vi "Handle Error.vi"(8 "error in (no error)":errorcluster, 11 "VHM-VNA_Hardware_Manager in":refnum<class "VHM-VNA_Hardware_Manager.lvclass">) -> (0 "error out":errorcluster, 2 "stop actor?":bool=TRUE, 3 "VHM-VNA_Hardware_Manager out":refnum<class "VHM-VNA_Hardware_Manager.lvclass">)   [LabVIEW 2020, in "VHM-VNA_Hardware_Manager.lvlib" / "VHM-VNA_Hardware_Manager.lvclass"]
doc: "(<B>Filename</B>: Actor Framework.lvlib:Actor.lvclass:Handle Error.vi)\n\nDefines how the actor handles an error that occurred while processing a message. By default, this method does nothing except stop the actor."
uses:
  VHM-VNA_Hardware_Manager.lvclass
  <vilib>/ActorFramework/Actor/Actor.lvclass
  common/features/CF-common_features.lvlib
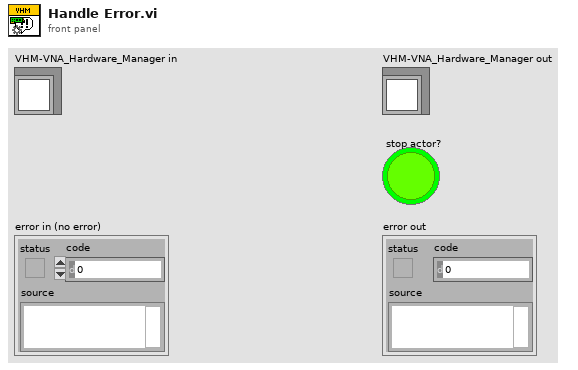
[diagram p1: front panel]
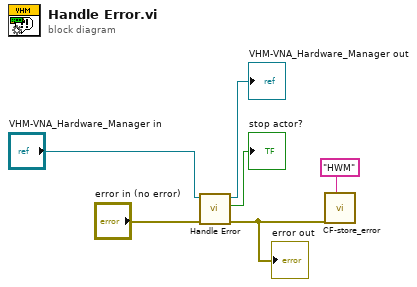
[diagram p0: block diagram]
diagram:
  n1 = call-parent "Handle Error.vi"("error in (no error)"="error in (no error)", "Actor in"="VHM-VNA_Hardware_Manager in") -> ("error out"=w2:errorcluster, "stop actor?"=→"stop actor?":bool, "Actor out"=→"VHM-VNA_Hardware_Manager out":refnum<class "VHM-VNA_Hardware_Manager.lvclass">)  [unwired: 7 in]
  "error out" <- w2
  n2 = call "CF-store_error.vi"("Location"="HWM", "error in (no error)"=w2) -> ()  [unwired: 10 in]
